vi "Get Cell Item From Index.vi"(8 "错误输入":errorcluster, 10 "Index":cluster{"Row":i32, "Col":i32}, 11 "Mlistbox Ref":refnum<vi>) -> (0 "错误输出":errorcluster, 2 "Item":string, 3 "Mlistbox Ref Dup":refnum<vi>)   [LabVIEW 2012, in "Mlistbox Tools.lvlib"]
uses:
  Mlistbox Tools.lvlib
  ListBox/Custom Type/Read and Write Mode.ctl
  Property/Set and Get ItemNames.vi
  ListBox/Listbox Tool.lvlib
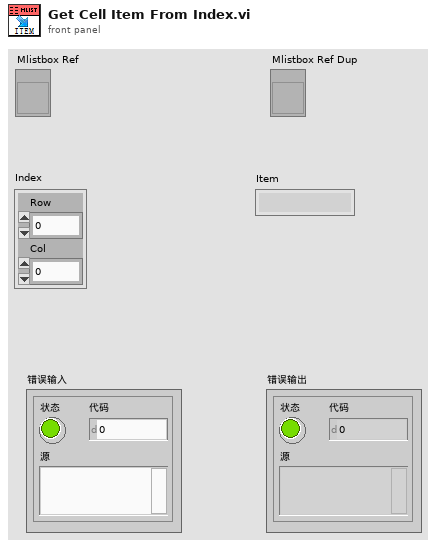
[diagram p1: front panel]
types:
  T1 = typedef "Listbox Tool.lvlib/Read and Write Mode.ctl" = enum16{"Read", "Write"}
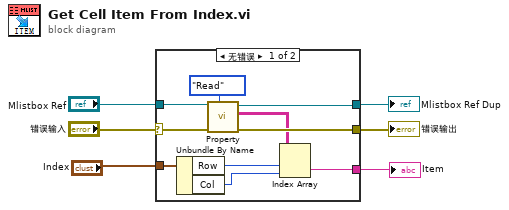
[diagram p0: block diagram]
diagram:
  n1 = case shown="无错误" "错误输入" {
    selector: "错误输入" -> [w14 w18]
    tunnel: [w12 w18] -> w5
    tunnel: "Mlistbox Ref" -> [w16 w17]
    tunnel: [w13 w17] -> w3
    tunnel: "Index" -> [w9 _]
    tunnel: [w10 _] -> w1
    frame No Error {
      n2 = Unbundle By Name(w9) -> ("Row"=w8:i32, "Col"=w7:i32)
      n3 = call-poly "Property.vi"("Mode"=Read_and_Write_Mode."Read", "错误输入"=w14, "Mlistbox Ref"=w16) -> ("错误输出"=w12:errorcluster, "ItemNames Out"=w11:string[][], "Mlistbox Ref Dup"=w13:refnum<vi>)  [unwired: 6 in]
      n4 = Index Array(array=w11, index (row)=w8, index (col)=w7) -> (element=w10:string)
    }
    frame Error {
    }
  }
  "Mlistbox Ref Dup" <- w3
  "错误输出" <- w5
  "Item" <- w1
